vi "initialize_fpga_usb.vi"(4 "error in":errorcluster, 6 "Baud Rate":u32=115200, 7 "Device Description":string="Ultracool FPGA") -> (0 "error out":errorcluster, 3 "Handle":u32)   [LabVIEW 2013, in "DDS9954_v2013.lvlib"]
uses:
  DDS9954_v2013.lvlib
panel:
  in  "Flow Control":u16(ring) items=["None"=0, "RTS-CTS"=256, "DTR-DSR"=512, "XOn-XOff"=1024]
  in  "Parity":u8(ring) items=["FT_PARITY_NONE", "FT_PARITY_ODD", "FT_PARITY_EVEN", "FT_PARITY_MARK", "FT_PARITY_SPACE"]
  in  "Stop Bits":u8(ring) items=["FT_STOP_BITS_1"=0, "FT_STOP_BITS_2"=2]
  in  "Word Length":u8(ring)=8 items=["FT_BITS_7"=7, "FT_BITS_8"=8]
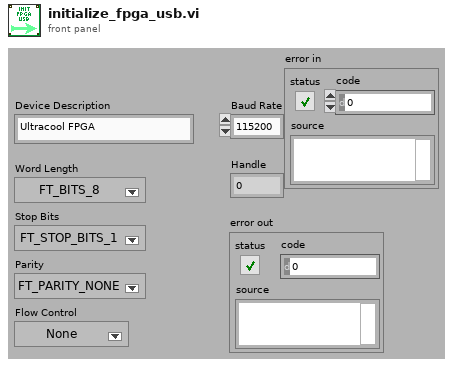
[diagram p1: front panel]
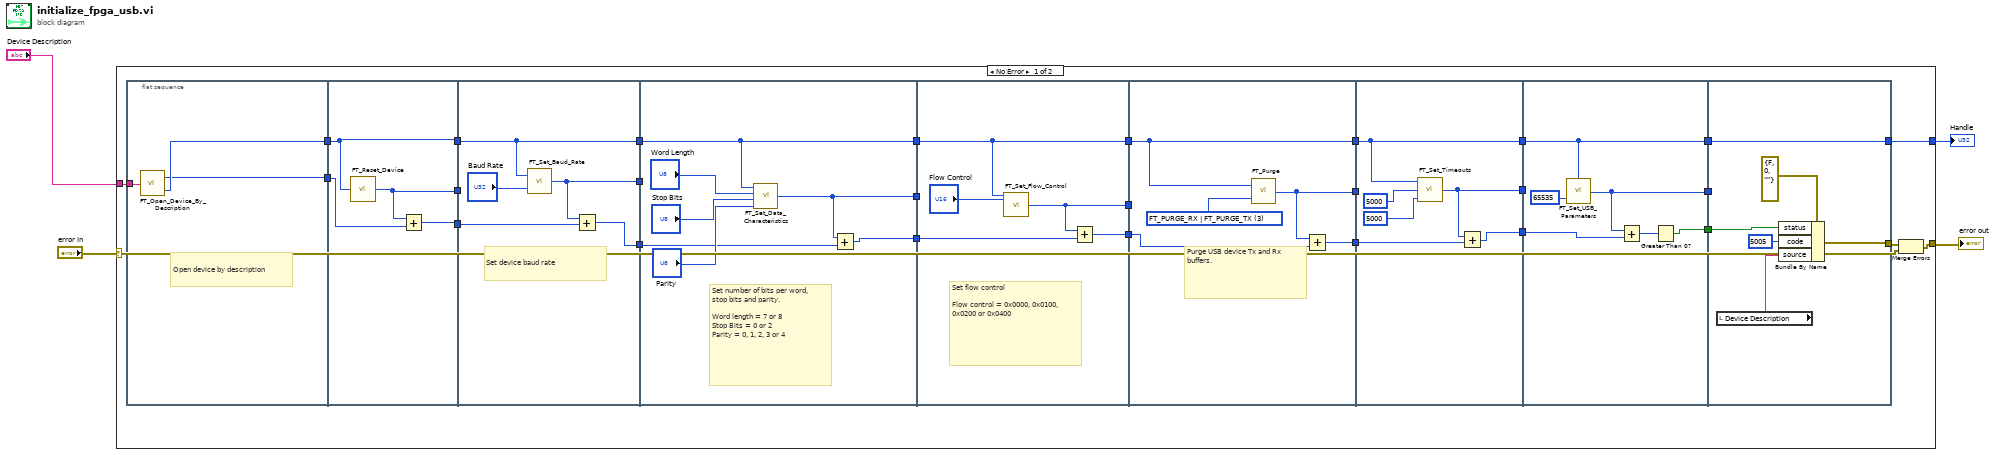
[diagram p0: block diagram]
diagram:
  n1 = case shown="No Error" "error in" {
    selector: "error in" -> [w5 w80]
    tunnel: [w9 _] -> w4
    tunnel: "Device Description" -> [w8 _]
    tunnel: [w6 w80] -> w2
    frame No Error {
      n2 = flat-sequence {
        tunnel: [w35] -> w32
        tunnel: w8 -> [w34]
        tunnel: [w33] -> w31
        tunnel: w32 -> [w39]
        tunnel: [w39] -> w30
        tunnel: [w38] -> w29
        tunnel: w31 -> [w37]
        tunnel: [w36] -> w28
        tunnel: w30 -> [w44]
        tunnel: [w44] -> w27
        tunnel: w29 -> [_]
        tunnel: [w42] -> w26
        tunnel: w28 -> [w41]
        tunnel: [w40] -> w25
        tunnel: w27 -> [w51]
        tunnel: [w51] -> w24
        tunnel: w26 -> [_]
        tunnel: [w46] -> w23
        tunnel: w25 -> [w47]
        tunnel: [w45] -> w22
        tunnel: w24 -> [w56]
        tunnel: [w56] -> w21
        tunnel: w23 -> [_]
        tunnel: [w54] -> w20
        tunnel: w22 -> [w53]
        tunnel: [w52] -> w19
        tunnel: w21 -> [w60]
        tunnel: [w60] -> w18
        tunnel: w20 -> [_]
        tunnel: [w59] -> w17
        tunnel: w19 -> [w58]
        tunnel: [w57] -> w16
        tunnel: w18 -> [w67]
        tunnel: [w67] -> w15
        tunnel: w17 -> [_]
        tunnel: [w64] -> w14
        tunnel: w16 -> [w63]
        tunnel: [w62] -> w13
        tunnel: w15 -> [w73]
        tunnel: w14 -> [_]
        tunnel: [w73] -> w12
        tunnel: [w71] -> w11
        tunnel: w13 -> [w70]
        tunnel: [w68] -> w10
        tunnel: [w79] -> w9
        tunnel: w12 -> [w79]
        tunnel: w11 -> [_]
        tunnel: w10 -> [w77]
        tunnel: [w74] -> w7
        frame #0 {
          # "Open device by description"
          n3 = call "FT_Open_Device_By_Description.vi"("Device Description"=w34) -> ("FT_Status"=w33:u32, "Handle"=w35:u32)
        }
        frame #1 {
          n4 = call "FT_Reset_Device.vi"("Handle"=w39) -> ("FT_Status"=w38:u32)
          n5 = Add(x=w38, y=w37) -> (x+y=w36:u32)
        }
        frame #2 {
          # "Set device baud rate"
          n6 = call "FT_Set_Baud_Rate.vi"("Baud Rate"="Baud Rate", "Handle"=w44) -> ("FT_Status"=w42:u32)
          n7 = Add(x=w42, y=w41) -> (x+y=w40:u32)
        }
        frame #3 {
          # "Set number of bits per word, stop bits and parity.\n\nWord length = 7 or 8\nStop Bits = 0 or 2\nParity = 0, 1, 2, 3 or 4"
          n8 = call "FT_Set_Data_Characteristics.vi"("Parity"="Parity", "Stop Bits"="Stop Bits", "Word Length"="Word Length", "Handle"=w51) -> ("FT_Status"=w46:u32)
          n9 = Add(x=w46, y=w47) -> (x+y=w45:u32)
        }
        frame #4 {
          # "Set flow control\n\nFlow control = 0x0000, 0x0100, 0x0200 or 0x0400"
          n10 = call "FT_Set_Flow_Control.vi"("Flow Control"="Flow Control", "Handle"=w56) -> ("FT_Status"=w54:u32)  [unwired: 2 in]
          n11 = Add(x=w54, y=w53) -> (x+y=w52:u32)
        }
        frame #5 {
          w61 = u32 3 items=["FT_PURGE_RX"=1, "FT_PURGE_TX"=2, "FT_PURGE_RX | FT_PURGE_TX"=3] ("Purge Flags")
          # "Purge USB device Tx and Rx buffers."
          n12 = call "FT_Purge.vi"("Purge Flags"=w61, "Handle"=w60) -> ("FT_Status"=w59:u32)
          n13 = Add(x=w59, y=w58) -> (x+y=w57:u32)
        }
        frame #6 {
          n14 = call "FT_Set_Timeouts.vi"("Write Timeout"=u32 5000, "Read Timeout"=u32 5000, "Handle"=w67) -> ("FT_Status"=w64:u32)
          n15 = Add(x=w64, y=w63) -> (x+y=w62:u32)
        }
        frame #7 {
          n16 = call "FT_Set_USB_Parameters.vi"("In Transfer Size"=u32 65535, "Handle"=w73) -> ("FT_Status"=w71:u32)
          n17 = Add(x=w71, y=w70) -> (x+y=w69:u32)
          n18 = Greater Than 0?(x=w69) -> (x > 0?=w68:bool)
        }
        frame #8 {
          n19 = local read "Device Description"() -> (w76:string)
          n20 = Bundle By Name(cluster=errorcluster {"status"=FALSE, "code"=0, "source"=""} ("error constant"), "status"=w77, "code"=5005, "source"=w76) -> (w74:errorcluster)
        }
      }
      n21 = Merge Errors(w7, w5) -> (w6:errorcluster)
    }
    frame Error {
    }
  }
  "Handle" <- w4
  "error out" <- w2
